vi "FPGA_Calibration.vi"() -> ()   [LabVIEW 2013]
uses:
  <vilib>/rvi/interface/nirviOpenFPGA/nirviOpenFPGA.xnode
  <vilib>/rvi/interface/nirviCloseFPGA/nirviCloseFPGA.xnode
  <vilib>/FPGAPlugInAG/Dynamic/niLvFpga_Close_Dynamic.vi
panel:
  in  "Reverse Winch Direction?":bool
  in  "Upper Winch Percent":dbl
  in  "Lower Winch Percent":dbl
  in  "Rudder Range (deg)":dbl=100.0
  in  "Rudder Trim":dbl(slide) scale=-20.0..20.0
  # "Change value to reset zero\nin order to make up for human error setting up"
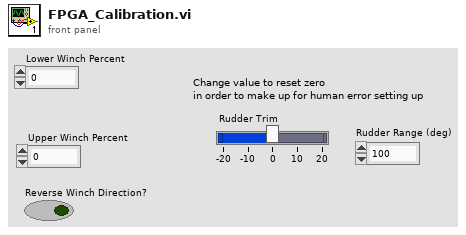
[diagram p1: front panel]
types:
  T1 = typedef "setpoints to boat.ctl" = cluster{"Sail Position":T2, "Rudder Angle":T3}
  T2 = typedef "sail setpt.ctl" = dbl
  T3 = typedef "rudder angle.ctl" = dbl
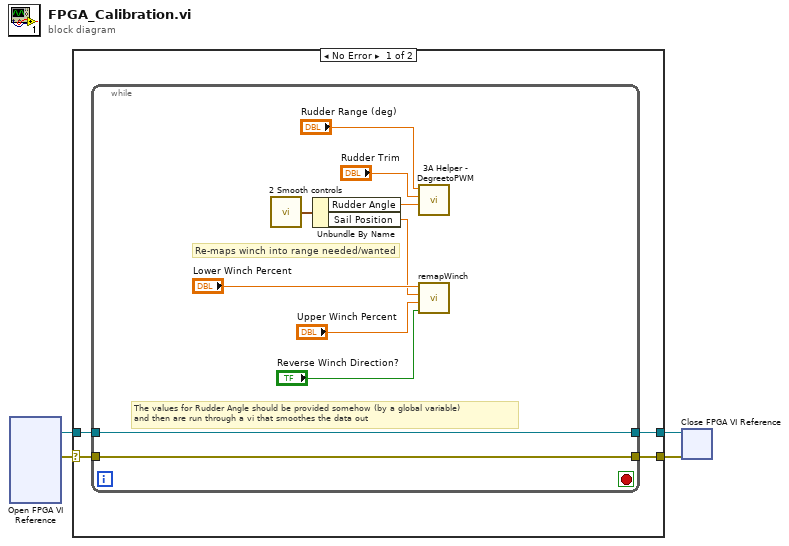
[diagram p0: block diagram]
diagram:
  n1 = xnode "Open FPGA VI Reference"() -> ("FPGA VI Reference Out"=w3:refnum<k20>, "error out"=w4:errorcluster)  [unwired: 2 in]
  n2 = case shown="No Error" w4 {
    selector: w4 -> [w6 _]
    tunnel: w3 -> [w8 _]
    tunnel: [w7 _] -> w2
    tunnel: [w5 _] -> w1
    frame No Error {
      n3 = while {
        tunnel: w8 -> [w11]
        tunnel: [w11] -> w7
        tunnel: w6 -> [w10]
        tunnel: [w10] -> w5
        stop <- _ stop-if-true
        # "Re-maps winch into range needed/wanted"
        # "The values for Rudder Angle should be provided somehow (by a global variable)\nand then are run through a vi that smoothes the data out"
        n4 = call "2 Smooth controls.vi"() -> ("Smoothed Setpoints out"=w14:T1)  [unwired: 5 in]
        n5 = Unbundle By Name(w14) -> ("Rudder Angle"=w13:T3, "Sail Position"=w12:T2)
        n6 = call "3A Helper - DegreetoPWM.vi"("Rudder Angle"=w13, "Rudder Trim"="Rudder Trim", "Rudder Range (deg)"="Rudder Range (deg)") -> ()  [unwired: 8 in, 1 out]
        n7 = call "remapWinch.vi"("Reverse Winch Direction?"="Reverse Winch Direction?", "Upper Winch Percent"="Upper Winch Percent", "Input Percent"=w12, "Lower Winch Percent"="Lower Winch Percent") -> ()  [unwired: 7 in, 1 out]
      }
    }
    frame Error {
      # "There is an error, will not continue"
    }
  }
  n8 = xnode "Close FPGA VI Reference"("FPGA VI Reference In"=w2, "error in"=w1) -> ()  [unwired: 1 out]
